vi "UsrProfiles-Default user.vi"(8 "error in (no error)":errorcluster) -> (0 "error out":errorcluster, 2 "Selected user's name":string, 3 "Default user selected":bool)   [LabVIEW 2020]
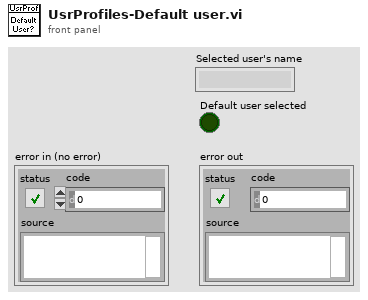
[diagram p1: front panel]
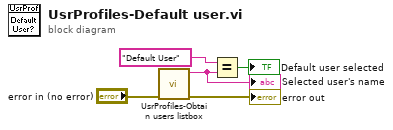
[diagram p0: block diagram]
diagram:
  n1 = call "UsrProfiles-Obtain users listbox.vi"("error in (no error)"="error in (no error)") -> ("error out"=→"error out":errorcluster, "Selected user's name"=w1:string)  [unwired: 7 in, 2 out]
  "Selected user's name" <- w1
  n2 = Equal?(x="Default User", y=w1) -> (x = y?=→"Default user selected":bool)
